vi "KE6221 -- Get Wave Ranging Mode.vi"(0 "Resource In":refnum<visa-resource-name>, 1 "Check For SCPI Errors? (T)":bool=TRUE, 11 "error in (no error)":errorcluster) -> (4 "Resource Out (dupl)":refnum<visa-resource-name>, 8 "Ranging Mode":T1, 15 "error out":errorcluster)   [LabVIEW 2019, in "Keithley 622x.lvlib"]
uses:
  Keithley 622x.lvlib
  Typedefs/KE6221 -- Wave Ranging Mode.ctl
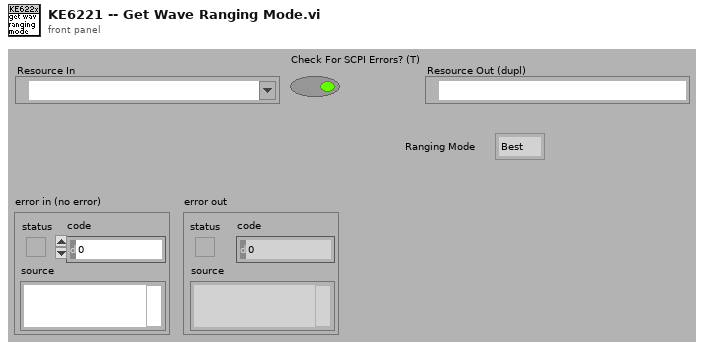
[diagram p1: front panel]
types:
  T1 = typedef "Keithley 622x.lvlib/KE6221 -- Wave Ranging Mode.ctl" = enum16{"Best", "Fixed"}
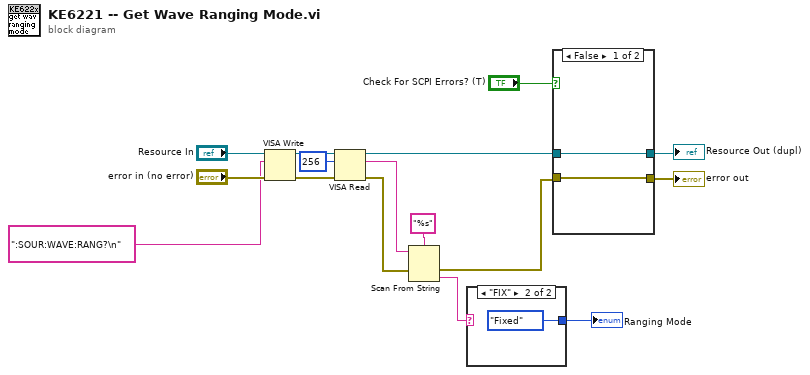
[diagram p0: block diagram]
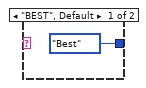
[diagram p2: hidden frame]
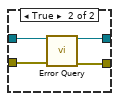
[diagram p3: hidden frame]
diagram:
  n1 = VISA Write(VISA resource name="Resource In", write buffer=":SOUR:WAVE:RANG?\n" ("format string"), error in (no error)="error in (no error)") -> (VISA resource name out=w10:refnum<visa-resource-name>, error out=w9:errorcluster)  [unwired: 1 out]
  n2 = VISA Read(VISA resource name=w10, byte count=u32 256, error in (no error)=w9) -> (VISA resource name out=w3:refnum<visa-resource-name>, read buffer=w5:string, error out=w7:errorcluster)  [unwired: 1 out]
  n3 = Scan From String(format string="%s", input string=w5, error in=w7) -> (error out=w4:errorcluster, output 1=w2:string)  [unwired: 2 in, 2 out]
  n4 = case shown="\"FIX\"" w2 {
    tunnel: [KE6221_--_Wave_Ranging_Mode."Best" ("Ranging Mode") KE6221_--_Wave_Ranging_Mode."Fixed" ("Ranging Mode")] -> w1
    frame "BEST", Default {
    }
    frame "FIX" {
    }
  }
  "Ranging Mode" <- w1
  n5 = case shown="False" "Check For SCPI Errors? (T)" {
    tunnel: w3 -> [w20 w24]
    tunnel: w4 -> [w19 w23]
    tunnel: [w19 w22] -> w12
    tunnel: [w20 w21] -> w13
    frame False {
    }
    frame True {
      n6 = call "Error Query.vi"("VISA Resource In"=w24, "error in (no error)"=w23) -> ("VISA Resource Out (dupl)"=w21:refnum<visa-resource-name>, "error out"=w22:errorcluster)  [unwired: 10 in, 2 out]
    }
  }
  "Resource Out (dupl)" <- w13
  "error out" <- w12
